vi "GetLoopParameters.vi"(8 "error in (no error)":errorcluster) -> (0 "error out":errorcluster, 3 "This VI":refnum<vi>)   [LabVIEW 2018]
uses:
  <vilib>/Utility/error.llb/DialogType.ctl
  <vilib>/Analysis/1siggen.llb/Ramp Pattern by Samples.vi
  Initialize References/Sequence Globals.vi
  Test Parameter Globals_1.0.0.vi
  <vilib>/Utility/file.llb/Write Delimited Spreadsheet (DBL).vi
  <vilib>/Utility/file.llb/Read Delimited Spreadsheet (string).vi
  <vilib>/Analysis/1siggen.llb/Ramp Pattern by Delta.vi
  Initialize References/Station References Global.vi
  Automated Tests/Tetra WAM/Tetra_Globals.vi
  <vilib>/Utility/file.llb/Write Delimited Spreadsheet (string).vi
  Test Result File Name Global.vi
  <vilib>/Analysis/NI_AALBase.lvlib
panel:
  out "VI Name":string
  out "test_param_path":path
  in  "STOP TEST":bool
  out "#of Iterations(str)":string
  out "Caption.Text":string
  out "Slide":dbl(slide) max=1608.0 step=1.0 scale=0.0..24.0
  out "# of iterations":i32=3
  out "count":dbl
  out "x-y 13":dbl
  out "x-y 12":dbl
  out "x-y 11":dbl
  out "x-y 10":dbl
  out "x-y 9":dbl
  out "x-y 8":dbl
  out "x-y 7":dbl
  out "x-y 6":dbl
  out "x-y 5":dbl
  out "x-y 4":dbl
  out "x-y 3":dbl
  out "x-y 2":dbl
  out "x-y":dbl
  out "Close vi":string="C:\\IdtATE\\Charactorization Tests\\F1200\\SParameter\\F1200_SP_Payload_10.0.0.0.vi"
  out "Test Parameters File":string caption="Test File:"
  out "F-format string":string
  out "Global SN":string="0"
  out "SN":string="15"
  in  "Use auto generated Directory/File Name (T)":bool=TRUE
  out "Test Results File Name":path=path "C:/IdtATE/Results/F1200-ZD_SP_CHAR/F1200-ZD_SP_CHAR_SN_0_131622.csv"
  out "Test Name":string="F1200-ZD_SP_CHAR"
  out "index of element":i32=2
  out "subarray":string[](array[string])=["", "", "TEST NAME", "SN", "", "KEY", "1", "1", "", "KEY", "1", "1", "1", "1", "1", "", "KEY", "3", "3", "-2", "-1", "-1", "-1", "-1", "-1", "", "KEY", "1", "1", "1", "1", "1", "1", "1", "1", "1", "1", "1", "1", "1", "1", "1", "1", "1", "1", "1", "1", "1", "1", "1", "1", "1", "1", "1", "1", "1", "1", "1", "1", "1", "1", "1", "1", "1", "1", "1", "1", "1", "1", "", ""]
  out "Payload vi":string="C:\\IdtATE\\Charactorization Tests\\F1200\\SParameter\\F1200_SP_Payload_10.0.0.0.vi"
  out "Setup vi":string="C:\\IdtATE\\Charactorization Tests\\F1200\\SParameter\\F1200_SP_Setup_10.0.0.0.vi"
  out "Computer Name":string="corpmxl0251xct"
  out "Outputs":string[](array[string])=["GAIN_CODE(8b Word)", "ICC(A)", "S11_30(mag)", "S11_30(ang)", "S21_30(mag)", "S21_30(ang)", "S12_30(mag)", "S12_30(ang)", "S22_30(mag)", "S22_30(ang)", "S11_50(mag)", "S11_50(ang)", "S21_50(mag)", "S21_50(ang)", "S12_50(mag)", "S12_50(ang)", "S22_50(mag)", "S22_50(ang)", "S11_80(mag)", "S11_80(ang)", "S21_80(mag)", "S21_80(ang)", "S12_80(mag)", "S12_80(ang)", "S22_80(mag)", "S22_80(ang)", "S11_100(mag)", "S11_100(ang)", "S21_100(mag)", "S21_100(ang)", "S12_100(mag)", "S12_100(ang)", "S22_100(mag)", "S22_100(ang)", "S11_120(mag)", "S11_120(ang)", "S21_120(mag)", "S21_120(ang)", "S12_120(mag)", "S12_120(ang)", "S22_120(mag)", "S22_120(ang)"]
  out "Output Keys":i32[](array[numeric])=[1, 1, 1, 1, 1, 1, 1, 1, 1, 1, 1, 1, 1, 1, 1, 1, 1, 1, 1, 1, 1, 1, 1, 1, 1, 1, 1, 1, 1, 1, 1, 1, 1, 1, 1, 1, 1, 1, 1, 1, 1, 1]
  out "Last Output Index":i32=68
  out "Loop Info":string[](array[string])=["LIST TEMP:19:-46:79", "LIST VCC:4.75:5:5.25", "RANGE GAIN[-1.25:22]0.25", "846"]
  out "!st Output Index":i32=27
  out "Loop Names":string[](array[string])=["TEMP", "VCC", "GAIN"]
  out "Loop Keys":i32[](array[numeric])=[3, 3, -2, -1, -1, -1, -1, -1]
  out "Const Names":string[](array[string])=["VNA_RECALL (reg)", "CAL_STD (text)", "CAL_FILE (path)", "SOAK_TIME (sec)", "LPT1 Base Address (reg)"]
  out "Const Values":string[](array[string])=["1", "thru", "", "300", "1110"]
  out "Const Keys":i32[](array[numeric])=[1, 1, 1, 1, 1]
  out "Vi Keys":i32[](array[numeric])=[1, 1]
  out "Vi List":string[](array[string])=["C:\\IdtATE\\Charactorization Tests\\F1200\\SParameter\\F1200_SP_Setup_10.0.0.0.vi", "C:\\IdtATE\\Charactorization Tests\\F1200\\SParameter\\F1200_SP_Payload_10.0.0.0.vi"]
  out "# of Const":i32=5
  out "Last Vi Sequence Index":i32=7
  out "1st Vi Sequence Index":i32=6
  out "Loop Values":string[][](array[string])=[["19", "-46", "79", "", "", "", "", "", "", "", "", "", "", "", "", "", "", "", "", "", "", "", "", "", "", "", "", "", "", "", "", "", "", "", "", "", "", "", "", "", "", "", "", "", "", "", "", "", "", "", "", "", "", "", "", "", "", "", "", "", "", "", "", "", "", "", "", "", "", "", "", "", "", "", "", "", "", "", "", "", "", "", "", "", "", "", "", "", "", "", "", "", "", ""], ["4.75", "5", "5.25", "", "", "", "", "", "", "", "", "", "", "", "", "", "", "", "", "", "", "", "", "", "", "", "", "", "", "", "", "", "", "", "", "", "", "", "", "", "", "", "", "", "", "", "", "", "", "", "", "", "", "", "", "", "", "", "", "", "", "", "", "", "", "", "", "", "", "", "", "", "", "", "", "", "", "", "", "", "", "", "", "", "", "", "", "", "", "", "", "", "", ""], ["-1.250000", "-1.000000", "-0.750000", "-0.500000", "-0.250000", "0.000000", "0.250000", "0.500000", "0.750000", "1.000000", "1.250000", "1.500000", "1.750000", "2.000000", "2.250000", "2.500000", "2.750000", "3.000000", "3.250000", "3.500000", "3.750000", "4.000000", "4.250000", "4.500000", "4.750000", "5.000000", "5.250000", "5.500000", "5.750000", "6.000000", "6.250000", "6.500000", "6.750000", "7.000000", "7.250000", "7.500000", "7.750000", "8.000000", "8.250000", "8.500000", "8.750000", "9.000000", "9.250000", "9.500000", "9.750000", "10.000000", "10.250000", "10.500000", "10.750000", "11.000000", "11.250000", "11.500000", "11.750000", "12.000000", "12.250000", "12.500000", "12.750000", "13.000000", "13.250000", "13.500000", "13.750000", "14.000000", "14.250000", "14.500000", "14.750000", "15.000000", "15.250000", "15.500000", "15.750000", "16.000000", "16.250000", "16.500000", "16.750000", "17.000000", "17.250000", "17.500000", "17.750000", "18.000000", "18.250000", "18.500000", "18.750000", "19.000000", "19.250000", "19.500000", "19.750000", "20.000000", "20.250000", "20.500000", "20.750000", "21.000000", "21.250000", "21.500000", "21.750000", "22.000000"]]
  out "Last Const Index":i32=14
  out "1st Loop  Index":i32=17
  out "1st  Const Index":i32=10
types:
  T1 = typedef "DialogType.ctl" = u16
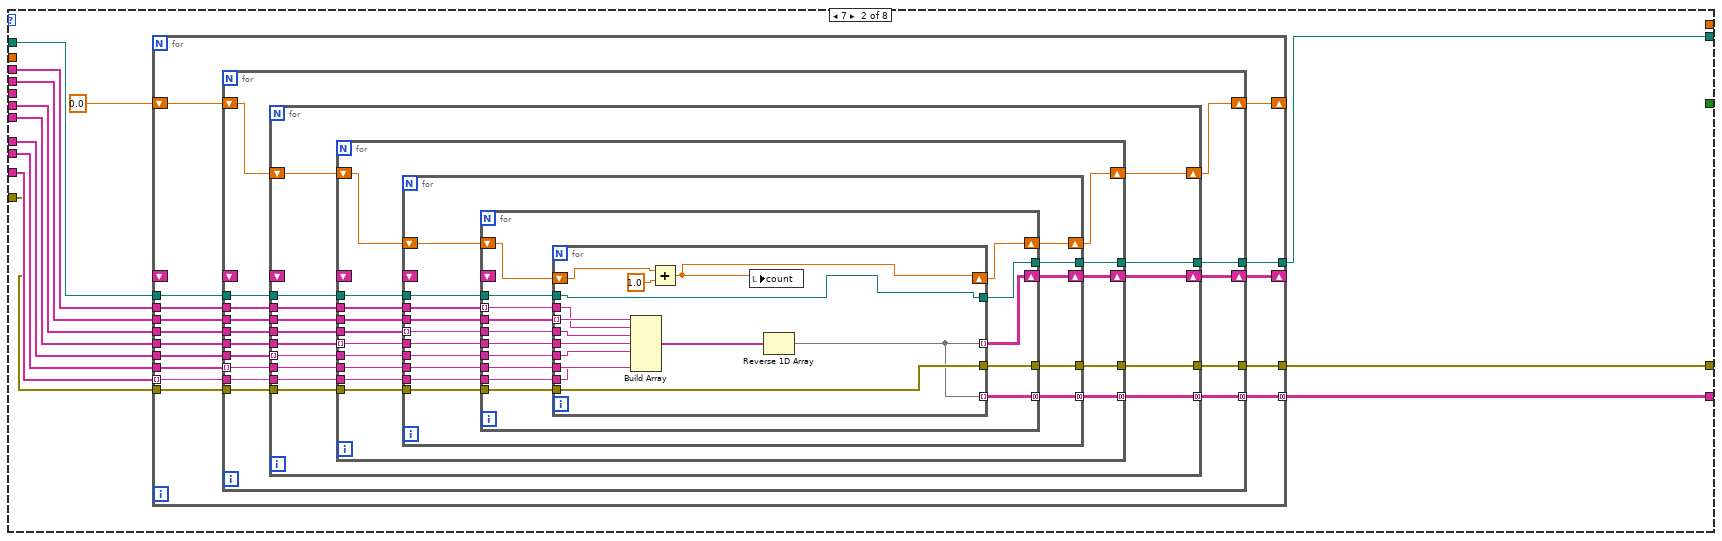
[diagram p3: hidden frame]
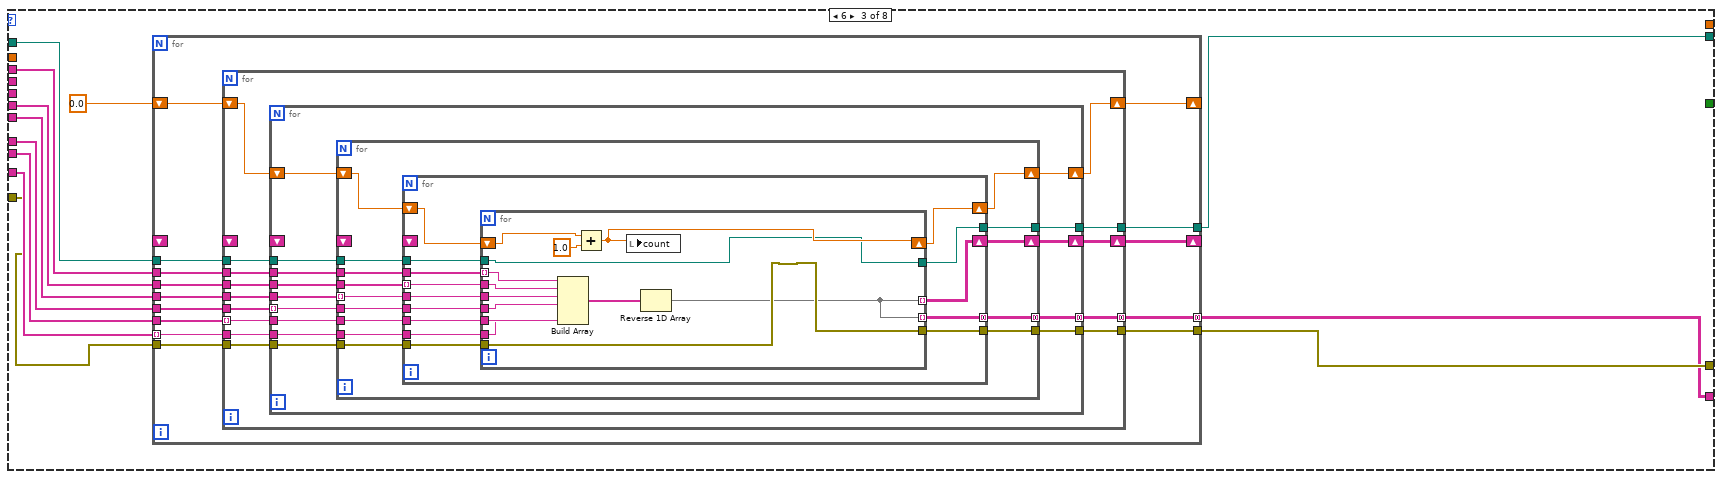
[diagram p4: hidden frame]
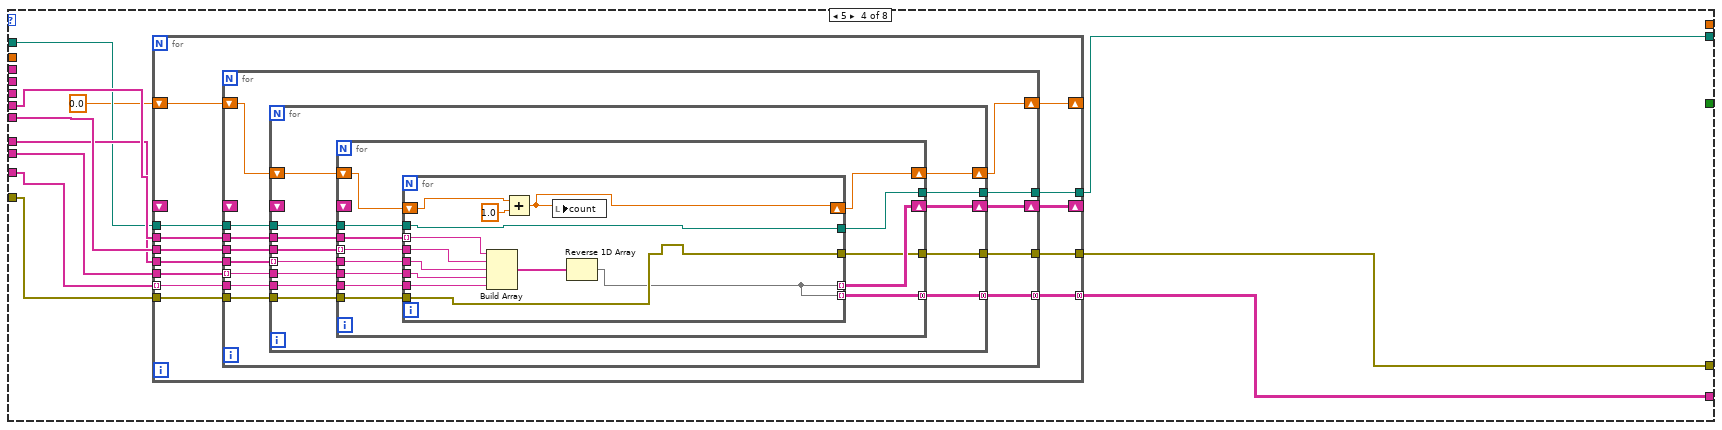
[diagram p5: hidden frame]
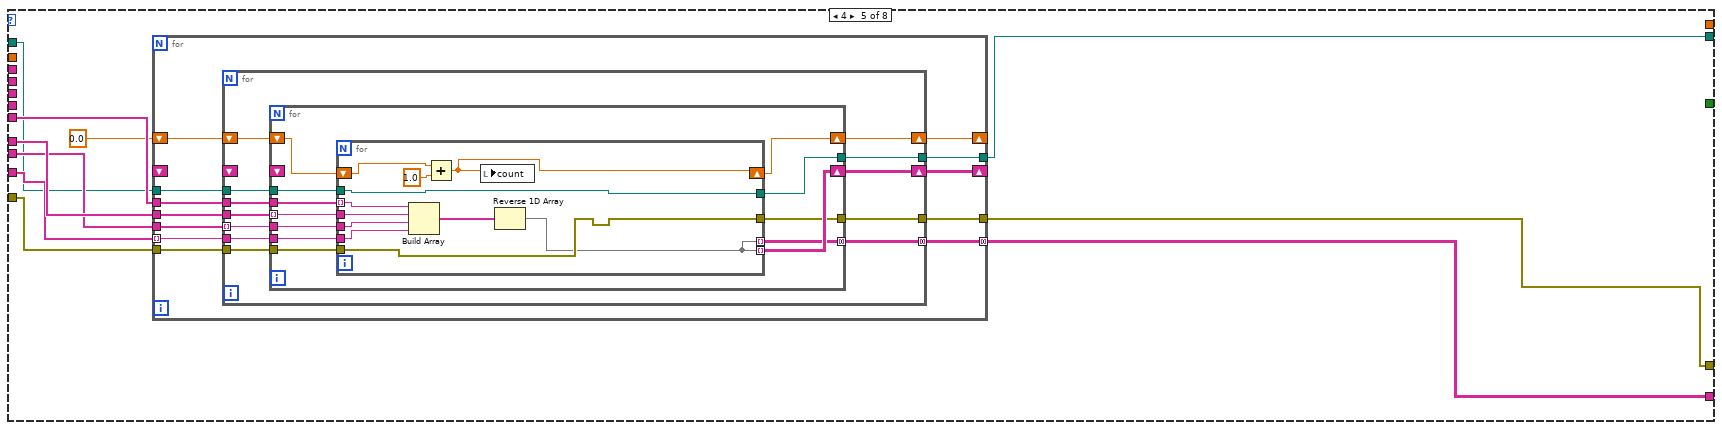
[diagram p6: hidden frame]
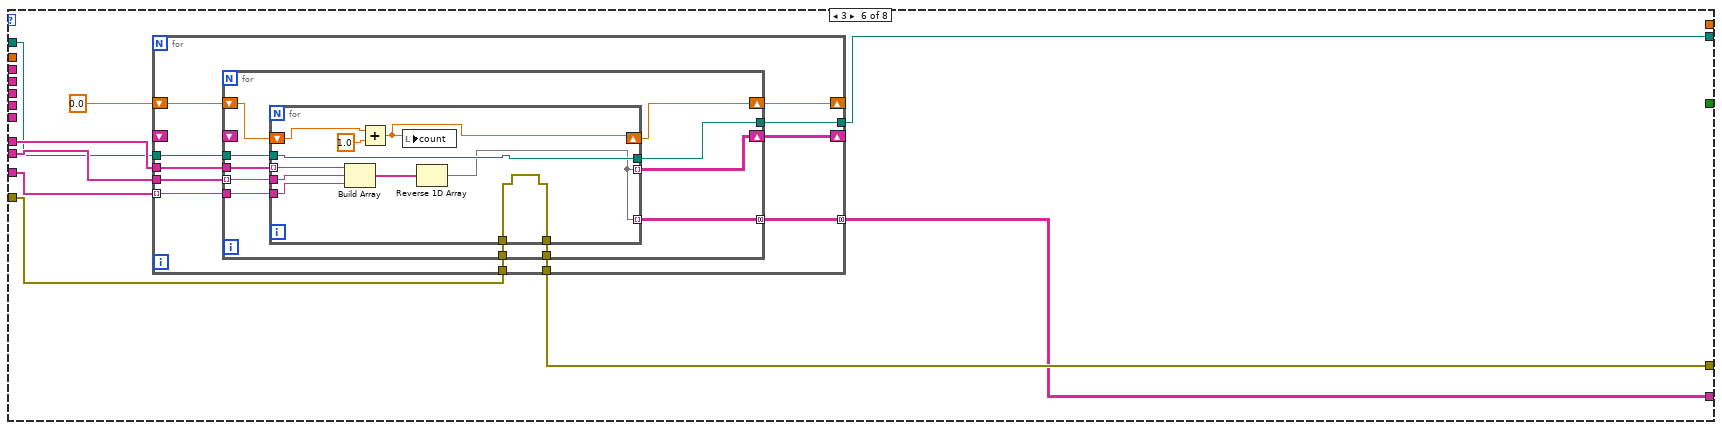
[diagram p7: hidden frame]
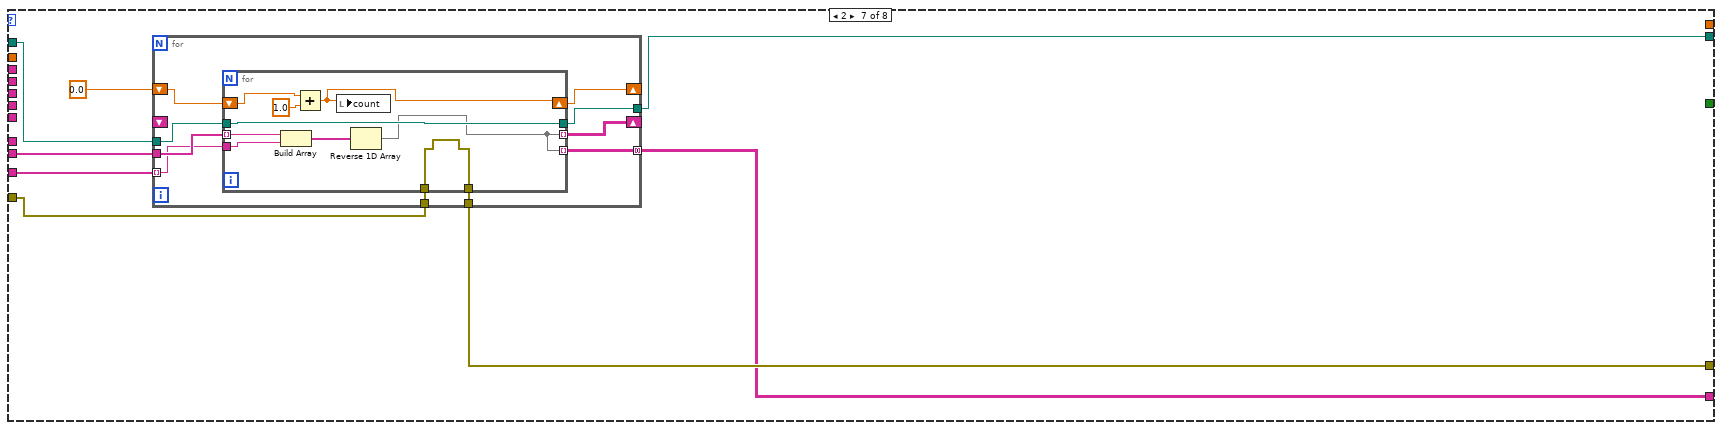
[diagram p8: hidden frame]
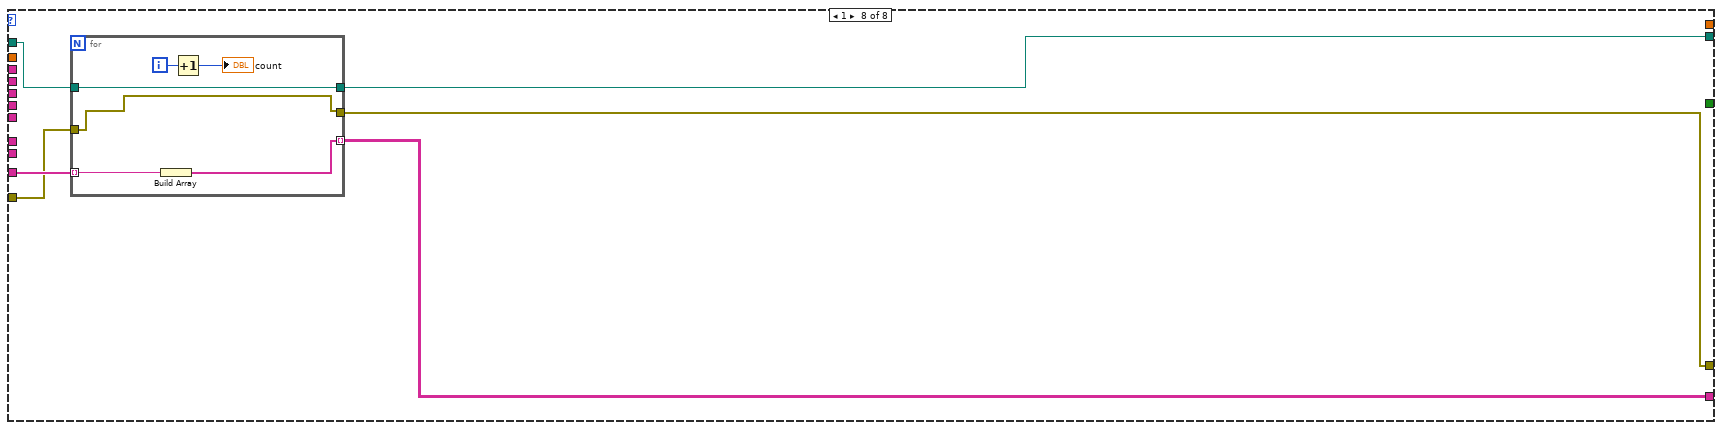
[diagram p9: hidden frame]
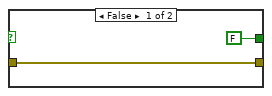
[diagram p13: hidden frame]
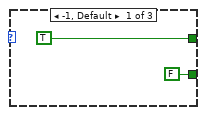
[diagram p16: hidden frame]
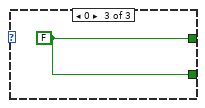
[diagram p17: hidden frame]
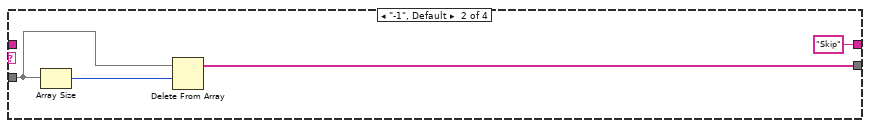
[diagram p18: hidden frame]
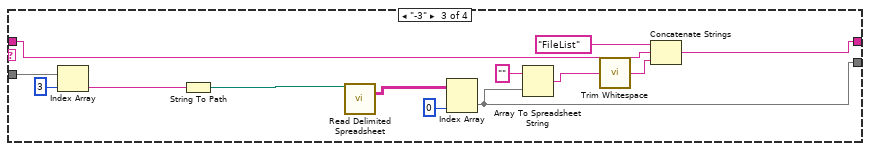
[diagram p19: hidden frame]
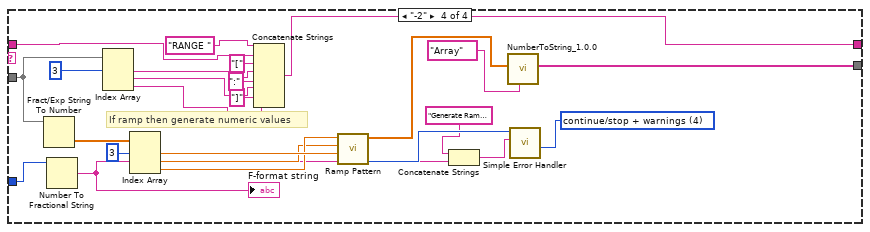
[diagram p20: hidden frame]
diagram:
  n1 = call <vilib>:"High Resolution Relative Seconds.vi"() -> ("relative seconds"=w35:dbl)
  n2 = flat-sequence {
    tunnel: [w86] -> w36
    tunnel: w35 -> [w85]
    tunnel: [w78] -> w19
    tunnel: [w97] -> w61
    tunnel: w36 -> [w117]
    tunnel: [w116] -> w34
    tunnel: w19 -> [w114]
    tunnel: [w108] -> w18
    tunnel: [w141] -> w72
    tunnel: [w139] -> w62
    tunnel: w61 -> [w139]
    tunnel: w34 -> [w137]
    tunnel: [w136] -> w33
    tunnel: w18 -> [w134]
    tunnel: [w131] -> w17
    tunnel: [w155] -> w60
    tunnel: w72 -> [w155]
    tunnel: w62 -> [_]
    tunnel: w33 -> [w149]
    tunnel: [w148] -> w32
    tunnel: w17 -> [w145]
    tunnel: [w144] -> w16
    tunnel: [w231] -> w66
    tunnel: w60 -> [w231]
    tunnel: w32 -> [w222]
    tunnel: [w221] -> w31
    tunnel: w16 -> [w219]
    tunnel: [w219] -> w10
    tunnel: w66 -> [w288]
    tunnel: [w288] -> w70
    tunnel: w31 -> [w276]
    tunnel: [w275] -> w30
    tunnel: [w273] -> w11
    tunnel: w10 -> [w273]
    tunnel: w70 -> [w325]
    tunnel: [w325] -> w71
    tunnel: w30 -> [w321]
    tunnel: [w320] -> w29
    tunnel: [w318] -> w12
    tunnel: w11 -> [w318]
    tunnel: [w358] -> w73
    tunnel: w71 -> [w351]
    tunnel: [w350] -> w69
    tunnel: [w349] -> w68
    tunnel: w29 -> [w348]
    tunnel: [w347] -> w28
    tunnel: [w345] -> w13
    tunnel: w12 -> [w345]
    tunnel: w68 -> [w379]
    tunnel: w69 -> [w380]
    tunnel: w73 -> [w382]
    tunnel: [w377] -> w59
    tunnel: [w382] -> w58
    tunnel: [w381] -> w57
    tunnel: [w377] -> w56
    tunnel: w28 -> [w376]
    tunnel: [w375] -> w27
    tunnel: [w373] -> w14
    tunnel: w13 -> [w373]
    tunnel: w59 -> [w463]
    tunnel: w58 -> [w462]
    tunnel: w57 -> [w461]
    tunnel: w56 -> [w459]
    tunnel: [w463] -> w46
    tunnel: [w462] -> w44
    tunnel: [w461] -> w42
    tunnel: w27 -> [w456]
    tunnel: [w455] -> w26
    tunnel: [w452] -> w15
    tunnel: w14 -> [w452]
    tunnel: w46 -> [w491]
    tunnel: [w491] -> w45
    tunnel: w44 -> [w490]
    tunnel: [w490] -> w43
    tunnel: w42 -> [w489]
    tunnel: [w489] -> w41
    tunnel: w26 -> [w476]
    tunnel: [w475] -> w25
    tunnel: w15 -> [w471]
    tunnel: [w470] -> w9
    tunnel: [w535] -> w65
    tunnel: [w536] -> w67
    tunnel: [w534] -> _
    tunnel: w45 -> [w534]
    tunnel: w43 -> [w536]
    tunnel: w41 -> [w535]
    tunnel: [w533] -> w54
    tunnel: [w532] -> w53
    tunnel: [w531] -> w52
    tunnel: [w530] -> w51
    tunnel: [w529] -> w50
    tunnel: [w528] -> w49
    tunnel: [w527] -> w48
    tunnel: [w526] -> w47
    tunnel: [w521] -> w55
    tunnel: w25 -> [w525]
    tunnel: [w524] -> w22
    tunnel: w9 -> [w519]
    tunnel: [w518] -> w8
    tunnel: [w517] -> w1
    frame #0 {
      n3 = global read "Sequence Globals.vi" "Stop Testing"() -> (w77:bool)
      n4 = control-ref of="Slide"() -> (w81:refnum<vi>)
      n5 = case shown="True" w77 {
        selector: w77 -> [_ w88]
        tunnel: "error in (no error)" -> [w87 w90]
        tunnel: [w87 w89] -> w75
        frame False {
        }
        frame True {
          n6 = global write "Sequence Globals.vi" "Stop Testing"(w88) -> ()
          n7 = flat-sequence {
            tunnel: w88 -> [w94]
            tunnel: [w94] -> w91
            tunnel: w90 -> [w93]
            tunnel: [w92] -> w89
            tunnel: w91 -> [w96]
            frame #0 {
              n8 = control-ref of="This VI"() -> (w95:refnum<vi>)
              n9 = invoke class="VI" method="FP.Close"(reference=w95, error in=w93) -> (error out=w92:errorcluster)  [unwired: 1 in, 2 out]
            }
            frame #1 {
              n10 = Stop(stop? (T)=w96) -> ()
            }
          }
        }
      }
      n11 = property on="Property Node" class="Slide (strict)"(reference=w81, "Caption.Text"="") -> ()  [unwired: 1 in, 2 out]
      n12 = call <vilib>:"High Resolution Relative Seconds.vi"() -> ("relative seconds"=w86:dbl)
      n13 = control-ref of="This VI"() -> (→"This VI":refnum<vi>)
      n14 = local write "STOP TEST"(FALSE ("STOP TEST")) -> ()
      n15 = Subtract(x=w86, y=w85) -> (x-y=→"x-y":dbl)
      n16 = call "Get_computername.vi"("error in (no error)"=w75) -> ("error out"=w78:errorcluster, "Computer Name"=w83:string)  [unwired: 9 in]
      "Computer Name" <- w83
      n17 = global write "Test Parameter Globals_1.0.0.vi" "Computer Name"(w83) -> ()
      "Slide" <- 0.0 ("Slide")
    }
    frame #1 {
      (unwired) path "C:/RageATE/Infrastructure/Test Parameters.tmp" ("file path (dialog if empty)")
      w99 = path "Infrastructure/Test Parameters.tmp" ("file path (dialog if empty)")
      # "Create temp parameter filename"
      n18 = global read "Sequence Globals.vi" "AppSupportPath"() -> (w110:path)
      n19 = global read "Sequence Globals.vi" "IsRuntime?"() -> (w113:bool)
      n20 = Strip Path(path=w99) -> (name=w112:string)  [unwired: 1 out]
      n21 = call <vilib>:"High Resolution Relative Seconds.vi"() -> ("relative seconds"=w116:dbl)
      n22 = global read "Sequence Globals.vi" "DevSupportPath"() -> (w101:path)
      n23 = Build Path(base path=w110, name or relative path=w112) -> (appended path=w111:path)
      n24 = Subtract(x=w116, y=w117) -> (x-y=→"x-y 2":dbl)
      n25 = property class="VI"() -> ("Name"=w104:string)  [unwired: 2 in, 2 out]
      "VI Name" <- w104
      n26 = Strip Path(path=w101) -> (stripped path=w100:path)  [unwired: 1 out]
      n27 = Build Path(base path=w100, name or relative path=w99) -> (appended path=w98:path)
      n28 = Select(t=w111, s=w113, f=w98) -> (s? t:f=w109:path)
      n29 = call-poly <vilib>:"Write Delimited Spreadsheet.vi"("file path (dialog if empty)"=w109, "append to file? (new file:F)"=FALSE, "error in (no error)"=w114, "delimiter (\\t)"="," ("delimiter (\\t)")) -> ("new file path (Not A Path if cancelled)"=w97:path, "error out"=w108:errorcluster)  [unwired: 10 in]
      "test_param_path" <- w97
      n30 = Path To String(path=w97) -> (string=w105:string)
      n31 = Format Into String(format string="%s in VI %s Cant be located", initial string="The File:  ", w105, w104) -> (resulting string=w103:string)  [unwired: 1 in, 1 out]
      n32 = call <vilib>:"Check if File or Folder Exists.vi"("error in (no error)"=w108, "path"=w97) -> ("file or folder exists?"=w102:bool)  [unwired: 7 in, 2 out]
      n33 = case shown="False" w102 {
        tunnel: w103 -> [w120 _]
        frame False {
          n34 = call "Display Message to User2"("Message"=w120) -> ()  [unwired: 9 in, 2 out]
        }
        frame True {
        }
      }
    }
    frame #2 {
      # "Get the test parameter file"
      n35 = global read "Test Parameter Globals_1.0.0.vi" "Test Parameters File"() -> (w123:path)
      n36 = Path To String(path=w123) -> (string=w125:string)
      n37 = property class="VI"() -> ("Name"=w126:string)  [unwired: 2 in, 2 out]
      n38 = call <vilib>:"Check if File or Folder Exists.vi"("path"=w123) -> ("file or folder exists?"=w127:bool)  [unwired: 8 in, 2 out]
      n39 = control-ref of="Test Parameters File"() -> (w133:refnum<vi>)
      n40 = Format Into String(format string="%s in VI %s Cant be located", initial string="The File:  ", w125, w126) -> (resulting string=w121:string)  [unwired: 1 in, 1 out]
      n41 = case shown="False" w127 {
        tunnel: w121 -> [w143 _]
        frame False {
          n42 = call "Display Message to User3"("Message"=w143) -> ()  [unwired: 9 in, 2 out]
        }
        frame True {
        }
      }
      n43 = call <vilib>:"High Resolution Relative Seconds.vi"() -> ("relative seconds"=w136:dbl)
      n44 = Path To String(path=w123) -> (string=w128:string)
      "Test Parameters File" <- w128
      n45 = Concatenate Strings("Test File: " ("string"), w128) -> (w129:string)
      n46 = Subtract(x=w136, y=w137) -> (x-y=→"x-y 3":dbl)
      n47 = call-poly <vilib>:"Read Delimited Spreadsheet.vi"("file path (dialog if empty)"=w123, "error in (no error)"=w134, "transpose? (F)"=FALSE ("transpose (no:F)")) -> ("all rows"=w138:string[][], "error out"=w132:errorcluster)  [unwired: 7 in, 4 out]
      n48 = property class="Str"(reference=w133, error in=w132, "Caption.Text"=w129) -> (error out=w131:errorcluster)  [unwired: 1 out]
      n49 = Delete From Array(array=w138, index (col)=0 ("disabled index (col)")) -> (array with subset deleted=w141:string[][])  [unwired: 2 in, 1 out]
    }
    frame #3 {
      w161 = 0 ("disabled index (col)")
      # "Generate Indices with a keyword search"
      n50 = To Upper Case(1:w155) -> (0:w164:string[][])
      n51 = call <vilib>:"High Resolution Relative Seconds.vi"() -> ("relative seconds"=w148:dbl)
      n52 = Subtract(x=w148, y=w149) -> (x-y=→"x-y 4":dbl)
      n53 = To Upper Case(1:"VI Sequence" ("element")) -> (0:w193:string)
      n54 = To Upper Case(1:"End Parameters" ("string")) -> (0:w175:string)
      n55 = To Upper Case(1:"Loop Parameters" ("element")) -> (0:w150:string)
      n56 = To Upper Case(1:"Outputs" ("string")) -> (0:w178:string)
      n57 = To Upper Case(1:"Input Constants" ("element")) -> (0:w191:string)
      n58 = Index Array(array=w155, index (col)=1 ("disabled index (col)")) -> (element=w165:string[])  [unwired: 1 in]
      n59 = Index Array(array=w164, index (col)=w161) -> (element=w146:string[])  [unwired: 1 in]
      "subarray" <- w146
      n60 = To Upper Case(1:w165) -> (0:w194:string[])
      n61 = To Upper Case(1:w165) -> (0:w176:string[])
      n62 = To Upper Case(1:w165) -> (0:w179:string[])
      n63 = To Upper Case(1:w165) -> (0:w166:string[])
      n64 = To Upper Case(1:w165) -> (0:w192:string[])
      n65 = To Upper Case(1:"TEST NAME" ("element")) -> (0:w151:string)
      n66 = To Upper Case(1:"SN" ("element")) -> (0:w157:string)
      n67 = Add(x=w161, y=1) -> (x+y=w154:i32)
      n68 = To Upper Case(1:w146) -> (0:w163:string[])
      n69 = Search 1D Array(1D array=w194, element=w193) -> (index of element=w183:i32)  [unwired: 1 in]
      n70 = Search 1D Array(1D array=w176, element=w175) -> (index of element=w173:i32)  [unwired: 1 in]
      n71 = Search 1D Array(1D array=w179, element=w178) -> (index of element=w170:i32)  [unwired: 1 in]
      n72 = Search 1D Array(1D array=w166, element=w191) -> (index of element=w181:i32)  [unwired: 1 in]
      n73 = Search 1D Array(1D array=w192, element=w150) -> (index of element=w182:i32)  [unwired: 1 in]
      n74 = To Upper Case(1:w146) -> (0:w156:string[])
      n75 = Search 1D Array(1D array=w163, element=w151) -> (index of element=w162:i32)  [unwired: 1 in]
      "index of element" <- w162
      n76 = Search 1D Array(1D array=w156, element=w157) -> (index of element=w153:i32)  [unwired: 1 in]
      n77 = Build Array(w183, w182, w181) -> (w180:i32[])
      n78 = Add(x=1, y=w183) -> (x+y=→"1st Vi Sequence Index":i32)
      n79 = Subtract(x=w173, y=2) -> (x-y=→"Last Output Index":i32)
      n80 = Add(x=w170, y=1) -> (x+y=→"!st Output Index":i32)
      n81 = Subtract(x=w181, y=2 ("x")) -> (x-y=→"Last Vi Sequence Index":i32)
      n82 = Add(x=w181, y=1) -> (x+y=w197:i32)
      "1st  Const Index" <- w197
      n83 = Add(x=0, y=w182) -> (x+y=w202:i32)
      n84 = for {
        tunnel: w180 -> [w212] mode=indexing
        tunnel: w145 -> [w208]
        tunnel: [w207] -> w144
        # "Check for Spreadsheet Errors"
        n85 = Equal?(x=w212, y=-1) -> (x = y?=w210:bool)
        n86 = case shown="True" w210 {
          tunnel: [FALSE ("OK") w217] -> w209
          tunnel: w208 -> [w213 w216]
          tunnel: [w213 w215] -> w207
          frame False {
          }
          frame True {
            n87 = call "Display Message to User"("error in (no error)"=w216) -> ("error out"=w215:errorcluster, "OK"=w217:bool)  [unwired: 9 in]
          }
        }
        n88 = Stop(stop? (T)=w209) -> ()
      }
      n89 = Subtract(x=w202, y=2) -> (x-y=w185:i32)
      "Last Const Index" <- w185
      n90 = Add(x=1, y=w202) -> (x+y=→"1st Loop  Index":i32)
      n91 = Subtract(x=w185, y=w197) -> (x-y=w199:i32)
      n92 = Index Array(array=w155, index (row)=w162, index (col)=w154) -> (element=w159:string)
      "Test Name" <- w159
      n93 = Index Array(array=w155, index (row)=w153, index (col)=w154) -> (element=→"SN":string)
      n94 = Add(x=w199, y=1) -> (x+y=→"# of Const":i32)
      n95 = global write "Test Parameter Globals_1.0.0.vi" "Test Name"(w159) -> ()
    }
    frame #4 {
      n96 = local read "Last Output Index"() -> (w226:i32)
      n97 = local read "!st Output Index"() -> (w227:i32)
      n98 = call <vilib>:"High Resolution Relative Seconds.vi"() -> ("relative seconds"=w221:dbl)
      n99 = Subtract(x=w221, y=w222) -> (x-y=→"x-y 5":dbl)
      n100 = Subtract(x=w226, y=w227) -> (x-y=w230:i32)
      n101 = Add(x=w230, y=1) -> (x+y=w228:i32)
      n102 = call-poly <vilib>:"Ramp Pattern.vi"("start"=w227, "end"=w226, "samples"=w228) -> ("Ramp Pattern"=w232:dbl[])  [unwired: 7 in, 1 out]
      n103 = for {
        tunnel: w231 -> [w249]
        tunnel: w232 -> [w242] mode=indexing
        tunnel: [w248] -> w225 mode=indexing
        tunnel: [w243] -> w218 mode=indexing
        tunnel: [w240] -> w224 mode=indexing
        n104 = Index Array(array=w249, index (row) #1=w242, index (col) #1=0 ("disabled index (col)"), index (row) #2=w242, index (col) #2=1 ("disabled index (col)"), index (row) #3=w242, index (col) #3=2 ("disabled index (col)")) -> (element #1=w245:string, element #2=w248:string, element #3=w240:string)
        n105 = Fract/Exp String To Number(string=w245, default (0 dbl)=0 ("default (0 DBL)")) -> (number=w243:i32)  [unwired: 2 in, 1 out]
      }
      "Output Keys" <- w218
      n106 = for {
        tunnel: w225 -> [w239] mode=indexing
        tunnel: w224 -> [w237] mode=indexing
        tunnel: [w235] -> w223 mode=indexing if=w233
        tunnel: w218 -> [w234] mode=indexing
        n107 = Concatenate Strings(w239, "(" ("string"), w237, ")" ("string")) -> (w235:string)
        n108 = Not Equal To 0?(x=w234) -> (x != 0?=w233:bool)
      }
      "Outputs" <- w223
    }
    frame #5 {
      # "Vi Keys\n0 = Dont run\n1= Run /FP open\n-1= Run /FP closed"
      n109 = local read "Last Vi Sequence Index"() -> (w292:i32)
      n110 = local read "1st Vi Sequence Index"() -> (w282:i32)
      n111 = Subtract(x=w292, y=w282) -> (x-y=w291:i32)
      n112 = call <vilib>:"High Resolution Relative Seconds.vi"() -> ("relative seconds"=w275:dbl)
      n113 = Add(x=w291, y=1) -> (x+y=w290:i32)
      n114 = Subtract(x=w275, y=w276) -> (x-y=→"x-y 6":dbl)
      n115 = call-poly <vilib>:"Ramp Pattern.vi"("start"=w282, "end"=w292, "samples"=w290) -> ("Ramp Pattern"=w287:dbl[])  [unwired: 7 in, 1 out]
      n116 = for {
        tunnel: w288 -> [w317]
        tunnel: w287 -> [w315] mode=indexing
        tunnel: [w316] -> w286 mode=indexing
        tunnel: [w310] -> w284 mode=indexing
        n117 = Index Array(array=w317, index (row) #1=w315, index (col) #1=0 ("disabled index (col)"), index (row) #2=w315, index (col) #2=2 ("disabled index (col)")) -> (element #1=w312:string, element #2=w316:string)
        n118 = Fract/Exp String To Number(string=w312, default (0 dbl)=0 ("default (0 DBL)")) -> (number=w310:i32)  [unwired: 2 in, 1 out]
      }
      "Vi List" <- w286
      "Vi Keys" <- w284
      n119 = global read "Sequence Globals.vi" "AppSupportPath"() -> (w261:path)
      n120 = global read "Sequence Globals.vi" "IsRuntime?"() -> (w259:bool)
      n121 = for {
        tunnel: w284 -> [w304] mode=indexing
        tunnel: [w303] -> w283 mode=indexing
        tunnel: [w302] -> w277 mode=indexing
        n122 = case shown="1" w304 {
          tunnel: [TRUE TRUE w309] -> w303
          tunnel: [FALSE TRUE w309] -> w302
          frame -1, Default {
          }
          frame 1 {
          }
          frame 0 {
            w309 = FALSE
          }
        }
      }
      n123 = Index Array(array=w286) -> (element #1=w285:string, element #2=w266:string, element #3=w281:string)  [unwired: 3 in]
      n124 = String To Path(string=w285) -> (path=w270:path)
      n125 = String To Path(string=w266) -> (path=w264:path)
      n126 = String To Path(string=w281) -> (path=w260:path)
      n127 = global write "Test Parameter Globals_1.0.0.vi" "Payload Path"(w264) -> ()
      n128 = global write "Test Parameter Globals_1.0.0.vi" "Close vi"(w260) -> ()
      n129 = global write "Test Parameter Globals_1.0.0.vi" "Setup Path"(w270) -> ()
      n130 = Strip Path(path=w260) -> (name=w262:string)  [unwired: 1 out]
      n131 = Strip Path(path=w270) -> (name=w271:string)  [unwired: 1 out]
      n132 = Build Path(base path=w261, name or relative path=w262) -> (appended path=w263:path)
      n133 = Strip Path(path=w264) -> (name=w268:string)  [unwired: 1 out]
      n134 = Build Path(base path=w261, name or relative path=w271) -> (appended path=w272:path)
      n135 = Build Path(base path=w261, name or relative path=w268) -> (appended path=w267:path)
      n136 = Select(t=w263, s=w259, f=w260) -> (s? t:f=w255:path)
      n137 = Index Array(array=w283) -> (element #1=w254:bool, element #2=w253:bool, element #3=w252:bool)  [unwired: 3 in]
      n138 = Path To String(path=w255) -> (string=→"Close vi":string)
      n139 = Index Array(array=w277) -> (element #1=w280:bool, element #2=w279:bool, element #3=w278:bool)  [unwired: 3 in]
      n140 = Select(t=w272, s=w259, f=w270) -> (s? t:f=w257:path)
      n141 = Select(t=w267, s=w259, f=w264) -> (s? t:f=w256:path)
      n142 = Path To String(path=w256) -> (string=→"Payload vi":string)
      n143 = Path To String(path=w257) -> (string=→"Setup vi":string)
      n144 = global write "Test Parameter Globals_1.0.0.vi" "Close vi"(w255) -> ()
      n145 = global write "Test Parameter Globals_1.0.0.vi" "Show Setup FP"(w280) -> ()
      n146 = global write "Test Parameter Globals_1.0.0.vi" "Show Payload FP"(w279) -> ()
      n147 = global write "Test Parameter Globals_1.0.0.vi" "Run Setup vi"(w254) -> ()
      n148 = global write "Test Parameter Globals_1.0.0.vi" "Run Payload vi"(w253) -> ()
      n149 = global write "Test Parameter Globals_1.0.0.vi" "Show Close FP"(w278) -> ()
      n150 = global write "Test Parameter Globals_1.0.0.vi" "Payload Path"(w256) -> ()
      n151 = global write "Test Parameter Globals_1.0.0.vi" "Run Close vi"(w252) -> ()
      n152 = global write "Test Parameter Globals_1.0.0.vi" "Setup Path"(w257) -> ()
      n153 = Build Array(w254, w253, w252) -> (w251:bool[])
      n154 = Build Array(w257, w256, w255) -> (w250:path[])
      n155 = for {
        tunnel: w251 -> [w297] mode=indexing
        tunnel: w250 -> [w294] mode=indexing
        n156 = local read "VI Name"() -> (w295:string)
        n157 = Format Into String(format string="The File < %s > cant be found\nVI : %s", w294, w295) -> (resulting string=w293:string)  [unwired: 2 in, 1 out]
        n158 = case shown="True" w297 {
          tunnel: w294 -> [_ w300]
          tunnel: w293 -> [_ w299]
          frame False {
          }
          frame True {
            n159 = call <vilib>:"Check if File or Folder Exists.vi"("path"=w300) -> ("file or folder exists?"=w298:bool)  [unwired: 8 in, 2 out]
            n160 = case shown="False" w298 {
              tunnel: w299 -> [w301 _]
              frame False {
                n161 = call "Display Message to User4"("Message"=w301) -> ()  [unwired: 9 in, 2 out]
              }
              frame True {
              }
            }
          }
        }
      }
    }
    frame #6 {
      # "Get the Input Constants"
      n162 = local read "Last Const Index"() -> (w327:i32)
      n163 = local read "1st  Const Index"() -> (w326:i32)
      n164 = local read "# of Const"() -> (w328:i32)
      n165 = call <vilib>:"High Resolution Relative Seconds.vi"() -> ("relative seconds"=w320:dbl)
      n166 = Subtract(x=w320, y=w321) -> (x-y=→"x-y 7":dbl)
      n167 = call-poly <vilib>:"Ramp Pattern.vi"("start"=w326, "end"=w327, "samples"=w328) -> ("Ramp Pattern"=w329:dbl[])  [unwired: 7 in, 1 out]
      n168 = for {
        tunnel: w325 -> [w344]
        tunnel: w329 -> [w337] mode=indexing
        tunnel: [w341] -> w324 mode=indexing
        tunnel: [w335] -> w323 mode=indexing
        tunnel: [w330] -> w322 mode=indexing
        n169 = Index Array(array=w344, index (row) #1=w337, index (col) #1=0 ("disabled index (col)"), index (row) #2=w337, index (col) #2=1 ("disabled index (col)"), index (row) #3=w337, index (col) #3=2 ("disabled index (col)"), index (row) #4=w337, index (col) #4=3 ("disabled index (col)")) -> (element #1=w340:string, element #2=w334:string, element #3=w332:string, element #4=w335:string)
        n170 = Concatenate Strings(w334, " (" ("string"), w332, ")" ("string")) -> (w330:string)
        n171 = Fract/Exp String To Number(string=w340, default (0 dbl)=0 ("default (0 DBL)")) -> (number=w341:i32)  [unwired: 2 in, 1 out]
      }
      "Const Keys" <- w324
      "Const Values" <- w323
      "Const Names" <- w322
    }
    frame #7 {
      # "Get the 8 Loops"
      # "Adjust the array size by counting -1 keys"
      n172 = local read "1st Loop  Index"() -> (w354:i32)
      n173 = Add(x=7.0 ("end"), y=w354) -> (x+y=w356:dbl)
      n174 = call-poly <vilib>:"Ramp Pattern.vi"("start"=w354, "end"=w356, "samples"=8 ("x")) -> ("Ramp Pattern"=w353:dbl[])  [unwired: 7 in, 1 out]
      n175 = call <vilib>:"High Resolution Relative Seconds.vi"() -> ("relative seconds"=w347:dbl)
      n176 = Subtract(x=w347, y=w348) -> (x-y=→"x-y 8":dbl)
      n177 = for {
        tunnel: w351 -> [w362]
        tunnel: w353 -> [w361] mode=indexing
        tunnel: [w366] -> w352 mode=indexing
        tunnel: [w364] -> w349 mode=indexing
        tunnel: [w360] -> w350 mode=indexing
        n178 = Index Array(array=w362, index (row) #1=w361, index (col) #1=0 ("disabled index (col)"), index (row) #2=w361, index (col) #2=1 ("disabled index (col)"), index (row) #3=w361) -> (element #1=w363:string, element #2=w364:string, element #3=w360:string[])  [unwired: 1 in]
        n179 = Fract/Exp String To Number(string=w363, default (0 dbl)=0 ("default (0 DBL)")) -> (number=w366:i32)  [unwired: 2 in, 1 out]
      }
      "Loop Keys" <- w352
      n180 = for {
        tunnel: [w371] -> w359 mode=indexing
        tunnel: w352 -> [w369] mode=indexing
        n181 = Not Equal?(x=w369, y=-1.0) -> (x != y?=w372:bool)
        n182 = Boolean To (0,1)(Boolean=w372) -> (0, 1=w371:i16)
      }
      n183 = Add Array Elements(numeric array=w359) -> (sum=w358:i16)
    }
    frame #8 {
      n184 = for {
        N: w382 -> [_]
        tunnel: w380 -> [w387] mode=indexing
        tunnel: [w386] -> w377 mode=indexing
        tunnel: w379 -> [w385] mode=indexing
        tunnel: [w385] -> w378 mode=indexing
        tunnel: [w384] -> w381 mode=indexing
        i -> [w383]
        n185 = stacked-sequence {
          tunnel: w387 -> [w394]
          tunnel: [w392] -> w386
          tunnel: w385 -> [w390]
          tunnel: [w389] -> w384
          tunnel: w383 -> [w388]
          frame #0 {
            n186 = Index Array(array=w394, index=0) -> (element=w391:string)
            n187 = case shown="\"1\".." w391 {
              selector: w391 -> [w401 _ _ _]
              tunnel: w394 -> [w402 w413 w426 w446]
              tunnel: [w395 w411 w420 w444] -> w392
              tunnel: [w399 "Skip" w421 w440] -> w389
              tunnel: w390 -> [w398 _ w418 w432]
              tunnel: w388 -> [_ _ _ w430]
              frame "1".. {
                n188 = Fract/Exp String To Number(string=w401) -> (number=w400:dbl)  [unwired: 3 in, 1 out]
                n189 = for {
                  N: w400 -> [_]
                  tunnel: w402 -> [w409]
                  tunnel: [w403] -> w395 mode=indexing
                  tunnel: [w404] -> w397 mode=indexing
                  i -> [w408]
                  n190 = Add(x=3, y=w408) -> (x+y=w406:i32)
                  n191 = Index Array(array=w409, index=w406) -> (element=w403:string)
                  n192 = Concatenate Strings(":" ("string"), w403) -> (w404:string)
                }
                n193 = Concatenate Strings("LIST ", w398, w397) -> (w399:string)
              }
              frame "-1", Default {
                n194 = Array Size(array=w413) -> (size(s)=w412:i32)
                n195 = Delete From Array(array=w413, length=w412) -> (array with subset deleted=w411:string[])  [unwired: 1 in, 1 out]
              }
              frame "-3" {
                n196 = Index Array(array=w426, index=3) -> (element=w424:string)
                n197 = String To Path(string=w424) -> (path=w425:path)
                n198 = call-poly <vilib>:"Read Delimited Spreadsheet.vi"("file path (dialog if empty)"=w425) -> ("all rows"=w414:string[][])  [unwired: 9 in, 5 out]
                n199 = Index Array(array=w414, index (col)=0 ("disabled index (col)")) -> (element=w420:string[])  [unwired: 1 in]
                n200 = Array To Spreadsheet String(array=w420, 3:"" ("format string")) -> (spreadsheet string=w416:string)  [unwired: 1 in]
                n201 = call <vilib>:"Trim Whitespace.vi"("string"=w416) -> ("trimmed string"=w415:string)  [unwired: 1 in]
                n202 = Concatenate Strings("FileList", w418, w415) -> (w421:string)
              }
              frame "-2" {
                w431 = T1 4 items=["no dialog", "OK message", "continue or stop message", "OK message + warnings", "continue/stop + warnings"] ("type of dialog (OK msg:1)")
                # "If ramp then generate numeric values"
                n203 = Fract/Exp String To Number(string=w446) -> (number=w451:dbl[])  [unwired: 3 in, 1 out]
                n204 = Number To Fractional String(number=w430) -> (F-format string=w428:string)  [unwired: 3 in]
                "F-format string" <- w428
                n205 = Index Array(array=w446, index #1=3 ("index")) -> (element #1=w438:string, element #2=w436:string, element #3=w434:string)  [unwired: 2 in]
                n206 = Index Array(array=w451, index #1=3 ("index")) -> (element #1=w450:dbl, element #2=w448:dbl, element #3=w449:dbl)  [unwired: 2 in]
                n207 = Concatenate Strings("RANGE " ("string"), w432, "[" ("string"), w438, ":" ("string"), w436, "]" ("string"), w434) -> (w440:string)
                n208 = call-poly <vilib>:"Ramp Pattern.vi"("start"=w450, "end"=w448, "delta"=w449) -> ("error"=w441:i32, "Ramp Pattern"=w443:dbl[])  [unwired: 6 in, 1 out]
                n209 = Concatenate Strings("Generate Ramp Pattern\nCheck Spreadsheet Ramp values at Index " ("error source (\" \")"), w428) -> (w427:string)
                n210 = call "NumberToString_1.0.0.vi"("Input Select"="Array", "Num (ary)"=w443) -> ("F-format string (ary)"=w444:string[])  [unwired: 8 in, 1 out]
                n211 = call <vilib>:"Simple Error Handler.vi"("error code (no error:0)"=w441, "error source (\" \")"=w427, "type of dialog (OK msg:1)"=w431) -> ()  [unwired: 2 in, 5 out]
              }
            }
          }
        }
      }
      "Loop Values" <- w377
      "Loop Names" <- w378
      n212 = call <vilib>:"High Resolution Relative Seconds.vi"() -> ("relative seconds"=w375:dbl)
      n213 = Subtract(x=w375, y=w376) -> (x-y=→"x-y 9":dbl)
    }
    frame #9 {
      n214 = global write "Test Parameter Globals_1.0.0.vi" "Test Parameters"(w459) -> ()
      n215 = local read "Const Values"() -> (w457:string[])
      n216 = local read "Loop Names"() -> (w453:string[])
      n217 = local read "Outputs"() -> (w460:string[])
      n218 = global write "Test Parameter Globals_1.0.0.vi" "Input Constants Out"(w457) -> ()
      n219 = call <vilib>:"High Resolution Relative Seconds.vi"() -> ("relative seconds"=w455:dbl)
      n220 = global write "Test Parameter Globals_1.0.0.vi" "Loop Names"(w453) -> ()
      n221 = Insert Into Array(array=w453, new element=w460) -> (w458:string[])  [unwired: 1 in]
      n222 = Subtract(x=w455, y=w456) -> (x-y=→"x-y 10":dbl)
      n223 = global write "Test Parameter Globals_1.0.0.vi" "Column Headers Global"(w458) -> ()
    }
    frame #10 {
      n224 = global read "Test Parameter Globals_1.0.0.vi" "User Prompt for SN (T)"() -> (w473:bool)
      n225 = call <vilib>:"High Resolution Relative Seconds.vi"() -> ("relative seconds"=w475:dbl)
      n226 = case shown="False" w473 {
        tunnel: [w492 w493] -> w479
        frame False {
          n227 = local read "SN"() -> (w492:string)
        }
        frame True {
          n228 = global read "Test Parameter Globals_1.0.0.vi" "Global SN"() -> (w493:string)
        }
      }
      "Global SN" <- w479
      n229 = Subtract(x=w475, y=w476) -> (x-y=→"x-y 11":dbl)
      n230 = global read "Test Parameter Globals_1.0.0.vi" "LOT ID"() -> (w465:string)
      n231 = global read "Station References Global.vi" "Test Station Information"() -> (w481:string)
      n232 = global read "Tetra_Globals.vi" "TestBench_ID"() -> (w468:string)
      n233 = global write "Test Parameter Globals_1.0.0.vi" "Global SN"(w479) -> ()
      n234 = local read "Payload vi"() -> (w482:string)
      n235 = local read "Setup vi"() -> (w485:string)
      n236 = Concatenate Strings(w479, "_" ("string"), w465) -> (w467:string)
      n237 = global read "Tetra_Globals.vi" "-ssid"() -> (w464:string)
      n238 = local read "Test Parameters File"() -> (w477:string)
      n239 = local read "Computer Name"() -> (w487:string)
      n240 = local read "Const Names"() -> (w484:string[])
      n241 = local read "Const Values"() -> (w483:string[])
      n242 = local read "Const Keys"() -> (w469:i32[])
      n243 = local read "Test Name"() -> (w486:string)
      n244 = call "GenerateHeaderAndFilename.vi"("Computer"=w487, "Instrument Information"=w481, "Test Name"=w486, "Payload vi Name"=w482, "Ssid"=w464, "Setup vi Name"=w485, "Test Parameter File Name"=w477, "Input Constants Keys"=w469, "SN"=w467, "Input Constants Names"=w484, "BenchId"=w468, "Input Constants Values"=w483) -> ("Header"=w472:string[], "Filename Path"=w480:path)  [unwired: 6 in]
      n245 = case shown="False" "Use auto generated Directory/File Name (T)" {
        tunnel: [w498 w514] -> w478
        tunnel: w480 -> [_ w509]
        tunnel: w472 -> [w497 w508]
        tunnel: w471 -> [w495 w506]
        tunnel: [w494 w505] -> w470
        frame False {
          n246 = Insert Into Array(array=w497, new element="" ("new element/subarray")) -> (w496:string[])  [unwired: 1 in]
          n247 = call-poly <vilib>:"Write Delimited Spreadsheet.vi"("1D data"=w496, "error in (no error)"=w495, "transpose? (no:F)"=TRUE, "delimiter (\\t)"="," ("delimiter (\\t)")) -> ("new file path (Not A Path if cancelled)"=w498:path, "error out"=w494:errorcluster)  [unwired: 10 in]
          n248 = call-poly <vilib>:"Write Delimited Spreadsheet.vi"("file path (dialog if empty)"=w498, "append to file? (new file:F)"=TRUE, "transpose? (no:F)"=TRUE, "delimiter (\\t)"="," ("delimiter (\\t)")) -> ()  [unwired: 10 in, 2 out]
        }
        frame True {
          n249 = Insert Into Array(array=w508, new element="" ("new element/subarray")) -> (w507:string[])  [unwired: 1 in]
          n250 = call-poly <vilib>:"Write Delimited Spreadsheet.vi"("file path (dialog if empty)"=w509, "1D data"=w507, "error in (no error)"=w506, "transpose? (no:F)"=TRUE, "delimiter (\\t)"="," ("delimiter (\\t)")) -> ("new file path (Not A Path if cancelled)"=w514:path, "error out"=w505:errorcluster)  [unwired: 9 in]
          n251 = call-poly <vilib>:"Write Delimited Spreadsheet.vi"("file path (dialog if empty)"=w514, "append to file? (new file:F)"=TRUE, "transpose? (no:F)"=TRUE, "delimiter (\\t)"="," ("delimiter (\\t)")) -> ()  [unwired: 10 in, 2 out]
        }
      }
      "Test Results File Name" <- w478
      n252 = global write "Test Result File Name Global.vi" "Test Results File Name"(w478) -> ()
    }
    frame #11 {
      w522 = "Generating Test Parameters File :"
      n253 = call "CleanUpArray.vi"("Ary In"=w534) -> ("Count"=w521:dbl, "Ary 1"=w526:string[], "Ary 2"=w527:string[], "Ary 3"=w528:string[], "Ary 4"=w529:string[], "Ary 5"=w530:string[], "Ary 6"=w531:string[], "Ary 7"=w532:string[], "Ary 8"=w533:string[])  [unwired: 18 in]
      "# of iterations" <- w521
      n254 = call <vilib>:"High Resolution Relative Seconds.vi"() -> ("relative seconds"=w524:dbl)
      n255 = Subtract(x=w524, y=w525) -> (x-y=→"x-y 12":dbl)
      n256 = global write "Test Parameter Globals_1.0.0.vi" "# of iterations"(w521) -> ()
      n257 = property on="Slide" class="Slide (strict)"(error in=w519, "Scale.Maximum"=w521, "Caption.Text"=w522) -> (error out=w518:errorcluster)  [unwired: 1 in, 1 out]
      n258 = Number To Decimal String(number=w521) -> (decimal integer string=→"#of Iterations(str)":string)  [unwired: 1 in]
      n259 = local read "test_param_path"() -> (w517:path)
      "Caption.Text" <- w522
    }
  }
  n260 = Array Size(array=w65) -> (size(s)=w64:i32)
  n261 = Number To Fractional String(number=w55, precision (6)=i16 0) -> (F-format string=w39:string)  [unwired: 2 in]
  n262 = case shown="8, Default" w67 {
    tunnel: w54 -> [w552 _ _ _ _ _ _ _]
    tunnel: w53 -> [w551 w707 _ _ _ _ _ _]
    tunnel: w52 -> [w550 w706 w823 _ _ _ _ _]
    tunnel: w51 -> [w549 w705 w822 w917 _ _ _ _]
    tunnel: w50 -> [w548 w704 w821 w916 w991 _ _ _]
    tunnel: w49 -> [w547 w703 w820 w915 w990 w1047 _ _]
    tunnel: w48 -> [w546 w702 w819 w914 w989 w1046 w1087 _]
    tunnel: w47 -> [w545 w701 w818 w913 w988 w1045 w1086 w1112]
    tunnel: [w544 w700 w817 w912 w987 w1044 w1085 w1111] -> w3
    tunnel: w1 -> [w543 w699 w816 w911 w986 w1043 w1084 w1110]
    tunnel: w22 -> [w542 _ _ _ _ _ _ _]
    tunnel: [w542 _ _ _ _ _ _ _] -> w23
    tunnel: [w540 _ _ _ _ _ _ _] -> w20
    tunnel: w8 -> [w538 w696 w814 w908 w984 w1040 w1082 w1109]
    tunnel: [w539 w697 w813 w909 w983 w1041 w1081 w1108] -> w6
    tunnel: [w537 w695 w812 w907 w982 w1039 w1080 w1107] -> w2
    frame 8, Default {
      n263 = for {
        tunnel: w552 -> [w569]
        tunnel: w551 -> [w568]
        tunnel: w550 -> [w567]
        tunnel: w549 -> [w566]
        tunnel: w548 -> [w565]
        tunnel: w547 -> [w564]
        tunnel: w546 -> [w563]
        tunnel: w545 -> [w562] mode=indexing
        shift-right: [w561] -> _
        shift-left: _ -> [_]
        tunnel: [w560] -> w544
        tunnel: w543 -> [w559]
        shift-right: [w557] -> _
        shift-left: 0.0 -> [w558]
        tunnel: [w556] -> w540
        tunnel: [w555] -> w539
        tunnel: w538 -> [w554]
        tunnel: [w553] -> w537 mode=concatenating
        stop <- w556 stop-if-true
        n264 = for {
          tunnel: w569 -> [w586]
          tunnel: w568 -> [w585]
          tunnel: w567 -> [w584]
          tunnel: w566 -> [w583]
          tunnel: w565 -> [w582]
          tunnel: w564 -> [w581]
          tunnel: w563 -> [w580] mode=indexing
          shift-right: [w579] -> w561
          shift-left: _ -> [_]
          tunnel: w562 -> [w578]
          tunnel: [w577] -> w560
          tunnel: w559 -> [w576]
          shift-right: [w574] -> w557
          shift-left: w558 -> [w575]
          tunnel: [w573] -> w556
          tunnel: [w572] -> w555
          tunnel: w554 -> [w571]
          tunnel: [w570] -> w553 mode=concatenating
          stop <- w573 stop-if-true
          n265 = for {
            tunnel: w586 -> [w603]
            tunnel: w585 -> [w602]
            tunnel: w584 -> [w601]
            tunnel: w583 -> [w600]
            tunnel: w582 -> [w599]
            tunnel: w581 -> [w598] mode=indexing
            shift-right: [w597] -> w579
            shift-left: _ -> [_]
            tunnel: w580 -> [w596]
            tunnel: w578 -> [w595]
            tunnel: [w594] -> w577
            tunnel: w576 -> [w593]
            shift-right: [w591] -> w574
            shift-left: w575 -> [w592]
            tunnel: [w590] -> w573
            tunnel: [w589] -> w572
            tunnel: w571 -> [w588]
            tunnel: [w587] -> w570 mode=concatenating
            stop <- w590 stop-if-true
            n266 = for {
              tunnel: w603 -> [w620]
              tunnel: w602 -> [w619]
              tunnel: w601 -> [w618]
              tunnel: w600 -> [w617]
              tunnel: w599 -> [w616] mode=indexing
              shift-right: [w615] -> w597
              shift-left: _ -> [_]
              tunnel: w598 -> [w614]
              tunnel: w596 -> [w613]
              tunnel: w595 -> [w612]
              tunnel: [w611] -> w594
              tunnel: w593 -> [w610]
              shift-right: [w608] -> w591
              shift-left: w592 -> [w609]
              tunnel: [w607] -> w590
              tunnel: [w606] -> w589
              tunnel: w588 -> [w605]
              tunnel: [w604] -> w587 mode=concatenating
              stop <- w607 stop-if-true
              n267 = for {
                tunnel: w620 -> [w637]
                tunnel: w619 -> [w636]
                tunnel: w618 -> [w635]
                tunnel: w617 -> [w634] mode=indexing
                shift-right: [w633] -> w615
                shift-left: _ -> [_]
                tunnel: w616 -> [w632]
                tunnel: w614 -> [w631]
                tunnel: w613 -> [w630]
                tunnel: w612 -> [w629]
                tunnel: [w628] -> w611
                tunnel: w610 -> [w627]
                shift-right: [w625] -> w608
                shift-left: w609 -> [w626]
                tunnel: [w624] -> w607
                tunnel: [w623] -> w606
                tunnel: w605 -> [w622]
                tunnel: [w621] -> w604 mode=concatenating
                stop <- w624 stop-if-true
                n268 = for {
                  tunnel: w637 -> [w654]
                  tunnel: w636 -> [w653]
                  tunnel: w635 -> [w652] mode=indexing
                  shift-right: [w651] -> w633
                  shift-left: _ -> [_]
                  tunnel: w634 -> [w650]
                  tunnel: w632 -> [w649]
                  tunnel: w631 -> [w648]
                  tunnel: w630 -> [w647]
                  tunnel: w629 -> [w646]
                  tunnel: [w645] -> w628
                  tunnel: w627 -> [w644]
                  shift-right: [w642] -> w625
                  shift-left: w626 -> [w643]
                  tunnel: [w641] -> w624
                  tunnel: [w640] -> w623
                  tunnel: w622 -> [w639]
                  tunnel: [w638] -> w621 mode=concatenating
                  stop <- w641 stop-if-true
                  n269 = for {
                    tunnel: w654 -> [w671]
                    shift-right: [w663] -> w651
                    shift-left: _ -> [_]
                    tunnel: w653 -> [w670] mode=indexing
                    tunnel: w652 -> [w669]
                    tunnel: w650 -> [w668]
                    tunnel: w649 -> [w667]
                    tunnel: w648 -> [w666]
                    tunnel: w647 -> [w665]
                    tunnel: w646 -> [w664]
                    tunnel: [w662] -> w645
                    tunnel: w644 -> [w661]
                    shift-right: [w659] -> w642
                    shift-left: w643 -> [w660]
                    tunnel: [w658] -> w641
                    tunnel: [w657] -> w640
                    tunnel: w639 -> [w656]
                    tunnel: [w655] -> w638 mode=concatenating
                    stop <- w658 stop-if-true
                    n270 = for {
                      tunnel: w671 -> [w694] mode=indexing
                      tunnel: w670 -> [w693]
                      tunnel: w669 -> [w692]
                      tunnel: w668 -> [w691]
                      tunnel: w667 -> [w690]
                      tunnel: w666 -> [w689]
                      tunnel: w665 -> [w688]
                      tunnel: w664 -> [w687]
                      tunnel: [w672] -> w663 mode=indexing
                      tunnel: [w673] -> w662
                      tunnel: w661 -> [w673]
                      shift-right: [w677] -> w659
                      shift-left: w660 -> [w684]
                      tunnel: ["STOP TEST"] -> w658
                      tunnel: [w675] -> w657
                      tunnel: w656 -> [w674]
                      tunnel: [w672] -> w655 mode=indexing
                      stop <- "STOP TEST" stop-if-true
                      n271 = Build Array(w694, w693, w692, w691, w690, w689, w688, w687) -> (w686:string[])
                      n272 = Add(x=w684, y=1.0) -> (x+y=w677:dbl)
                      n273 = local write "count"(w677) -> ()
                      n274 = local write "Slide"(w677) -> ()
                      n275 = local read "#of Iterations(str)"() -> (w680:string)
                      n276 = Reverse 1D Array(array=w686) -> (reversed array=w672:string[])
                      n277 = local read "Caption.Text"() -> (w682:string)
                      n278 = Number To Decimal String(number=w677) -> (decimal integer string=w681:string)  [unwired: 1 in]
                      n279 = Concatenate Strings(w682, w681, " of " ("string"), w680, " Iterations" ("string")) -> (w683:string)
                      n280 = property on="Slide" class="Slide (strict)"(error in=w674, "Caption.Text"=w683) -> (error out=w675:errorcluster)  [unwired: 1 in, 1 out]
                    }
                  }
                }
              }
            }
          }
        }
      }
    }
    frame 7 {
      n281 = for {
        tunnel: w707 -> [w722]
        tunnel: w706 -> [w721]
        tunnel: w705 -> [w720]
        tunnel: w704 -> [w719]
        tunnel: w703 -> [w718]
        tunnel: w702 -> [w717]
        shift-right: [w716] -> _
        shift-left: _ -> [_]
        tunnel: w701 -> [w715] mode=indexing
        tunnel: [w714] -> w700
        tunnel: w699 -> [w713]
        shift-right: [w712] -> _
        shift-left: 0.0 -> [w711]
        tunnel: [w710] -> w697
        tunnel: w696 -> [w709]
        tunnel: [w708] -> w695 mode=concatenating
        n282 = for {
          tunnel: w722 -> [w737]
          tunnel: w721 -> [w736]
          tunnel: w720 -> [w735]
          tunnel: w719 -> [w734]
          tunnel: w718 -> [w733]
          shift-right: [w732] -> w716
          shift-left: _ -> [_]
          tunnel: w717 -> [w731] mode=indexing
          tunnel: w715 -> [w730]
          tunnel: [w729] -> w714
          tunnel: w713 -> [w728]
          shift-right: [w726] -> w712
          shift-left: w711 -> [w727]
          tunnel: [w725] -> w710
          tunnel: w709 -> [w724]
          tunnel: [w723] -> w708 mode=concatenating
          n283 = for {
            tunnel: w737 -> [w752]
            tunnel: w736 -> [w751]
            tunnel: w735 -> [w750]
            tunnel: w734 -> [w749]
            shift-right: [w748] -> w732
            shift-left: _ -> [_]
            tunnel: w733 -> [w747] mode=indexing
            tunnel: w731 -> [w746]
            tunnel: w730 -> [w745]
            tunnel: [w744] -> w729
            tunnel: w728 -> [w743]
            shift-right: [w741] -> w726
            shift-left: w727 -> [w742]
            tunnel: [w740] -> w725
            tunnel: w724 -> [w739]
            tunnel: [w738] -> w723 mode=concatenating
            n284 = for {
              tunnel: w752 -> [w767]
              tunnel: w751 -> [w766]
              tunnel: w750 -> [w765]
              shift-right: [w764] -> w748
              shift-left: _ -> [_]
              tunnel: w749 -> [w763] mode=indexing
              tunnel: w747 -> [w762]
              tunnel: w746 -> [w761]
              tunnel: w745 -> [w760]
              tunnel: [w759] -> w744
              tunnel: w743 -> [w758]
              shift-right: [w756] -> w741
              shift-left: w742 -> [w757]
              tunnel: [w755] -> w740
              tunnel: w739 -> [w754]
              tunnel: [w753] -> w738 mode=concatenating
              n285 = for {
                tunnel: w767 -> [w782]
                tunnel: w766 -> [w781]
                shift-right: [w780] -> w764
                shift-left: _ -> [_]
                tunnel: w765 -> [w779] mode=indexing
                tunnel: w763 -> [w778]
                tunnel: w762 -> [w777]
                tunnel: w761 -> [w776]
                tunnel: w760 -> [w775]
                tunnel: [w774] -> w759
                tunnel: w758 -> [w773]
                shift-right: [w771] -> w756
                shift-left: w757 -> [w772]
                tunnel: [w770] -> w755
                tunnel: w754 -> [w769]
                tunnel: [w768] -> w753 mode=concatenating
                n286 = for {
                  shift-right: [w790] -> w780
                  shift-left: _ -> [_]
                  tunnel: w782 -> [w797]
                  tunnel: w781 -> [w796] mode=indexing
                  tunnel: w779 -> [w795]
                  tunnel: w778 -> [w794]
                  tunnel: w777 -> [w793]
                  tunnel: w776 -> [w792]
                  tunnel: w775 -> [w791]
                  tunnel: [w789] -> w774
                  tunnel: w773 -> [w788]
                  shift-right: [w786] -> w771
                  shift-left: w772 -> [w787]
                  tunnel: [w785] -> w770
                  tunnel: w769 -> [w784]
                  tunnel: [w783] -> w768 mode=concatenating
                  n287 = for {
                    tunnel: w797 -> [w811] mode=indexing
                    tunnel: w796 -> [w810]
                    tunnel: w795 -> [w809]
                    tunnel: w794 -> [w808]
                    tunnel: w793 -> [w807]
                    tunnel: w792 -> [w806]
                    tunnel: w791 -> [w805]
                    tunnel: [w798] -> w790 mode=indexing
                    tunnel: [w799] -> w789
                    tunnel: w788 -> [w799]
                    shift-right: [w801] -> w786
                    shift-left: w787 -> [w802]
                    tunnel: [w800] -> w785
                    tunnel: w784 -> [w800]
                    tunnel: [w798] -> w783 mode=indexing
                    n288 = Build Array(w811, w810, w809, w808, w807, w806, w805) -> (w804:string[])
                    n289 = Add(x=w802, y=1.0) -> (x+y=w801:dbl)
                    n290 = local write "count"(w801) -> ()
                    n291 = Reverse 1D Array(array=w804) -> (reversed array=w798:string[])
                  }
                }
              }
            }
          }
        }
      }
    }
    frame 6 {
      n292 = for {
        tunnel: w823 -> [w837]
        tunnel: w822 -> [w836]
        tunnel: w821 -> [w835]
        tunnel: w820 -> [w834]
        shift-right: [w833] -> _
        shift-left: _ -> [_]
        tunnel: w819 -> [w832]
        tunnel: w818 -> [w831] mode=indexing
        tunnel: [w830] -> w817
        tunnel: w816 -> [w829]
        shift-right: [w827] -> _
        shift-left: 0.0 -> [w828]
        tunnel: w814 -> [w826]
        tunnel: [w825] -> w813
        tunnel: [w824] -> w812 mode=concatenating
        n293 = for {
          tunnel: w837 -> [w851]
          tunnel: w836 -> [w850]
          tunnel: w835 -> [w849]
          shift-right: [w848] -> w833
          shift-left: _ -> [_]
          tunnel: w834 -> [w847]
          tunnel: w832 -> [w846] mode=indexing
          tunnel: w831 -> [w845]
          tunnel: [w844] -> w830
          tunnel: w829 -> [w843]
          shift-right: [w841] -> w827
          shift-left: w828 -> [w842]
          tunnel: w826 -> [w840]
          tunnel: [w839] -> w825
          tunnel: [w838] -> w824 mode=concatenating
          n294 = for {
            tunnel: w851 -> [w865]
            tunnel: w850 -> [w864]
            shift-right: [w863] -> w848
            shift-left: _ -> [_]
            tunnel: w849 -> [w862]
            tunnel: w847 -> [w861] mode=indexing
            tunnel: w846 -> [w860]
            tunnel: w845 -> [w859]
            tunnel: [w858] -> w844
            tunnel: w843 -> [w857]
            shift-right: [w855] -> w841
            shift-left: w842 -> [w856]
            tunnel: w840 -> [w854]
            tunnel: [w853] -> w839
            tunnel: [w852] -> w838 mode=concatenating
            n295 = for {
              tunnel: w865 -> [w879]
              shift-right: [w878] -> w863
              shift-left: _ -> [_]
              tunnel: w864 -> [w877]
              tunnel: w862 -> [w876] mode=indexing
              tunnel: w861 -> [w875]
              tunnel: w860 -> [w874]
              tunnel: w859 -> [w873]
              tunnel: [w872] -> w858
              tunnel: w857 -> [w871]
              shift-right: [w869] -> w855
              shift-left: w856 -> [w870]
              tunnel: w854 -> [w868]
              tunnel: [w867] -> w853
              tunnel: [w866] -> w852 mode=concatenating
              n296 = for {
                shift-right: [w887] -> w878
                shift-left: _ -> [_]
                tunnel: w879 -> [w893]
                tunnel: w877 -> [w892] mode=indexing
                tunnel: w876 -> [w891]
                tunnel: w875 -> [w890]
                tunnel: w874 -> [w889]
                tunnel: w873 -> [w888]
                tunnel: [w886] -> w872
                tunnel: w871 -> [w885]
                shift-right: [w883] -> w869
                shift-left: w870 -> [w884]
                tunnel: w868 -> [w882]
                tunnel: [w881] -> w867
                tunnel: [w880] -> w866 mode=concatenating
                n297 = for {
                  tunnel: w893 -> [w906] mode=indexing
                  tunnel: w892 -> [w905]
                  tunnel: w891 -> [w904]
                  tunnel: w890 -> [w903]
                  tunnel: w889 -> [w902]
                  tunnel: w888 -> [w901]
                  tunnel: [w894] -> w887 mode=indexing
                  tunnel: [w895] -> w886
                  tunnel: w885 -> [w895]
                  shift-right: [w897] -> w883
                  shift-left: w884 -> [w898]
                  tunnel: w882 -> [w896]
                  tunnel: [w896] -> w881
                  tunnel: [w894] -> w880 mode=indexing
                  n298 = Build Array(w906, w905, w904, w903, w902, w901) -> (w900:string[])
                  n299 = Add(x=w898, y=1.0) -> (x+y=w897:dbl)
                  n300 = local write "count"(w897) -> ()
                  n301 = Reverse 1D Array(array=w900) -> (reversed array=w894:string[])
                }
              }
            }
          }
        }
      }
    }
    frame 5 {
      n302 = for {
        tunnel: w917 -> [w930]
        tunnel: w916 -> [w929]
        shift-right: [w928] -> _
        shift-left: _ -> [_]
        tunnel: w915 -> [w927]
        tunnel: w914 -> [w926]
        tunnel: w913 -> [w925] mode=indexing
        tunnel: [w924] -> w912
        tunnel: w911 -> [w923]
        shift-right: [w921] -> _
        shift-left: 0.0 -> [w922]
        tunnel: [w920] -> w909
        tunnel: w908 -> [w919]
        tunnel: [w918] -> w907 mode=concatenating
        n303 = for {
          tunnel: w930 -> [w943]
          shift-right: [w942] -> w928
          shift-left: _ -> [_]
          tunnel: w929 -> [w941]
          tunnel: w927 -> [w940]
          tunnel: w926 -> [w939] mode=indexing
          tunnel: w925 -> [w938]
          tunnel: [w937] -> w924
          tunnel: w923 -> [w936]
          shift-right: [w934] -> w921
          shift-left: w922 -> [w935]
          tunnel: [w933] -> w920
          tunnel: w919 -> [w932]
          tunnel: [w931] -> w918 mode=concatenating
          n304 = for {
            shift-right: [w956] -> w942
            shift-left: _ -> [_]
            tunnel: w943 -> [w955]
            tunnel: w941 -> [w954]
            tunnel: w940 -> [w953] mode=indexing
            tunnel: w939 -> [w952]
            tunnel: w938 -> [w951]
            tunnel: [w950] -> w937
            tunnel: w936 -> [w949]
            shift-right: [w948] -> w934
            shift-left: w935 -> [w947]
            tunnel: [w946] -> w933
            tunnel: w932 -> [w945]
            tunnel: [w944] -> w931 mode=concatenating
            n305 = for {
              shift-right: [w964] -> w956
              shift-left: _ -> [_]
              tunnel: w955 -> [w969]
              tunnel: w954 -> [w968] mode=indexing
              tunnel: w953 -> [w967]
              tunnel: w952 -> [w966]
              tunnel: w951 -> [w965]
              tunnel: [w963] -> w950
              tunnel: w949 -> [w962]
              shift-right: [w961] -> w948
              shift-left: w947 -> [w960]
              tunnel: [w959] -> w946
              tunnel: w945 -> [w958]
              tunnel: [w957] -> w944 mode=concatenating
              n306 = for {
                tunnel: w969 -> [w981] mode=indexing
                tunnel: w968 -> [w980]
                tunnel: w967 -> [w979]
                tunnel: w966 -> [w978]
                tunnel: w965 -> [w977]
                tunnel: [w970] -> w964 mode=indexing
                tunnel: [w972] -> w963
                tunnel: w962 -> [w972]
                shift-right: [w973] -> w961
                shift-left: w960 -> [w974]
                tunnel: [w971] -> w959
                tunnel: w958 -> [w971]
                tunnel: [w970] -> w957 mode=indexing
                n307 = Build Array(w981, w980, w979, w978, w977) -> (w976:string[])
                n308 = Add(x=w974, y=1.0) -> (x+y=w973:dbl)
                n309 = local write "count"(w973) -> ()
                n310 = Reverse 1D Array(array=w976) -> (reversed array=w970:string[])
              }
            }
          }
        }
      }
    }
    frame 4 {
      n311 = for {
        shift-right: [w1003] -> _
        shift-left: _ -> [_]
        tunnel: w991 -> [w1002]
        tunnel: w990 -> [w1001]
        tunnel: w989 -> [w1000]
        tunnel: w988 -> [w999] mode=indexing
        tunnel: [w998] -> w987
        tunnel: w986 -> [w997]
        shift-right: [w995] -> _
        shift-left: 0.0 -> [w996]
        tunnel: w984 -> [w994]
        tunnel: [w993] -> w983
        tunnel: [w992] -> w982 mode=concatenating
        n312 = for {
          shift-right: [w1015] -> w1003
          shift-left: _ -> [_]
          tunnel: w1002 -> [w1014]
          tunnel: w1001 -> [w1013]
          tunnel: w1000 -> [w1012] mode=indexing
          tunnel: w999 -> [w1011]
          tunnel: [w1010] -> w998
          tunnel: w997 -> [w1009]
          shift-right: [w1007] -> w995
          shift-left: w996 -> [w1008]
          tunnel: w994 -> [w1006]
          tunnel: [w1005] -> w993
          tunnel: [w1004] -> w992 mode=concatenating
          n313 = for {
            shift-right: [w1023] -> w1015
            shift-left: _ -> [_]
            tunnel: w1014 -> [w1027]
            tunnel: w1013 -> [w1026] mode=indexing
            tunnel: w1012 -> [w1025]
            tunnel: w1011 -> [w1024]
            tunnel: [w1022] -> w1010
            tunnel: w1009 -> [w1021]
            shift-right: [w1019] -> w1007
            shift-left: w1008 -> [w1020]
            tunnel: w1006 -> [w1018]
            tunnel: [w1017] -> w1005
            tunnel: [w1016] -> w1004 mode=concatenating
            n314 = for {
              tunnel: w1027 -> [w1038] mode=indexing
              tunnel: w1026 -> [w1037]
              tunnel: w1025 -> [w1036]
              tunnel: w1024 -> [w1035]
              tunnel: [w1028] -> w1023 mode=indexing
              tunnel: [w1029] -> w1022
              tunnel: w1021 -> [w1029]
              shift-right: [w1033] -> w1019
              shift-left: w1020 -> [w1032]
              tunnel: w1018 -> [w1030]
              tunnel: [w1030] -> w1017
              tunnel: [w1028] -> w1016 mode=indexing
              n315 = Build Array(w1038, w1037, w1036, w1035) -> (w1034:string[])
              n316 = Add(x=w1032, y=1.0) -> (x+y=w1033:dbl)
              n317 = local write "count"(w1033) -> ()
              n318 = Reverse 1D Array(array=w1034) -> (reversed array=w1028:string[])
            }
          }
        }
      }
    }
    frame 3 {
      n319 = for {
        shift-right: [w1058] -> _
        shift-left: _ -> [_]
        tunnel: w1047 -> [w1057]
        tunnel: w1046 -> [w1056]
        tunnel: w1045 -> [w1055] mode=indexing
        tunnel: [w1054] -> w1044
        tunnel: w1043 -> [w1053]
        shift-right: [w1051] -> _
        shift-left: 0.0 -> [w1052]
        tunnel: [w1050] -> w1041
        tunnel: w1040 -> [w1049]
        tunnel: [w1048] -> w1039 mode=concatenating
        n320 = for {
          shift-right: [w1066] -> w1058
          shift-left: _ -> [_]
          tunnel: w1057 -> [w1069]
          tunnel: w1056 -> [w1068] mode=indexing
          tunnel: w1055 -> [w1067]
          tunnel: [w1065] -> w1054
          tunnel: w1053 -> [w1064]
          shift-right: [w1062] -> w1051
          shift-left: w1052 -> [w1063]
          tunnel: [w1061] -> w1050
          tunnel: w1049 -> [w1060]
          tunnel: [w1059] -> w1048 mode=concatenating
          n321 = for {
            tunnel: w1069 -> [w1079] mode=indexing
            tunnel: w1068 -> [w1078]
            tunnel: w1067 -> [w1077]
            tunnel: [w1070] -> w1066 mode=indexing
            tunnel: [w1072] -> w1065
            tunnel: w1064 -> [w1072]
            shift-right: [w1073] -> w1062
            shift-left: w1063 -> [w1074]
            tunnel: [w1071] -> w1061
            tunnel: w1060 -> [w1071]
            tunnel: [w1070] -> w1059 mode=indexing
            n322 = Build Array(w1079, w1078, w1077) -> (w1076:string[])
            n323 = Add(x=w1074, y=1.0) -> (x+y=w1073:dbl)
            n324 = local write "count"(w1073) -> ()
            n325 = Reverse 1D Array(array=w1076) -> (reversed array=w1070:string[])
          }
        }
      }
    }
    frame 2 {
      n326 = for {
        shift-right: [w1095] -> _
        shift-left: _ -> [_]
        tunnel: w1087 -> [w1097]
        tunnel: w1086 -> [w1096] mode=indexing
        tunnel: [w1094] -> w1085
        tunnel: w1084 -> [w1093]
        shift-right: [w1091] -> _
        shift-left: 0.0 -> [w1092]
        tunnel: w1082 -> [w1090]
        tunnel: [w1089] -> w1081
        tunnel: [w1088] -> w1080 mode=concatenating
        n327 = for {
          tunnel: w1097 -> [w1106] mode=indexing
          tunnel: w1096 -> [w1105]
          tunnel: [w1098] -> w1095 mode=indexing
          tunnel: [w1099] -> w1094
          tunnel: w1093 -> [w1099]
          shift-right: [w1101] -> w1091
          shift-left: w1092 -> [w1103]
          tunnel: w1090 -> [w1100]
          tunnel: [w1100] -> w1089
          tunnel: [w1098] -> w1088 mode=indexing
          n328 = Build Array(w1106, w1105) -> (w1104:string[])
          n329 = Add(x=w1103, y=1.0) -> (x+y=w1101:dbl)
          n330 = local write "count"(w1101) -> ()
          n331 = Reverse 1D Array(array=w1104) -> (reversed array=w1098:string[])
        }
      }
    }
    frame 1 {
      n332 = for {
        tunnel: w1112 -> [w1118] mode=indexing
        tunnel: [w1117] -> w1107 mode=indexing
        tunnel: [w1113] -> w1111
        tunnel: w1110 -> [w1113]
        tunnel: w1109 -> [w1114]
        tunnel: [w1114] -> w1108
        i -> [w1116]
        n333 = Build Array(w1118) -> (w1117:string[])
        n334 = Increment(x=w1116) -> (x+1=→"count":i32)
      }
    }
  }
  n335 = Concatenate Strings(w39, "Iterations" ("string")) -> (w37:string)
  n336 = Insert Into Array(array=w65, index=w64, new element=w37) -> (w40:string[])
  "Loop Info" <- w40
  n337 = global write "Test Parameter Globals_1.0.0.vi" "Loop Info"(w40) -> ()
  n338 = call <vilib>:"High Resolution Relative Seconds.vi"() -> ("relative seconds"=w24:dbl)
  n339 = case shown="True" w20 {
    selector: w20 -> [_ w1120]
    tunnel: w20 -> [_ w1123]
    tunnel: w6 -> [w1119 w1122]
    tunnel: [w1119 w1121] -> w7
    frame False {
    }
    frame True {
      n340 = global write "Sequence Globals.vi" "Stop Testing"(w1120) -> ()
      n341 = flat-sequence {
        tunnel: w1123 -> [w1127]
        tunnel: [w1127] -> w1124
        tunnel: w1122 -> [w1126]
        tunnel: [w1125] -> w1121
        tunnel: w1124 -> [w1129]
        frame #0 {
          n342 = control-ref of="This VI"() -> (w1128:refnum<vi>)
          n343 = invoke class="VI" method="FP.Close"(reference=w1128, error in=w1126) -> (error out=w1125:errorcluster)  [unwired: 1 in, 2 out]
        }
        frame #1 {
          n344 = Stop(stop? (T)=w1129) -> ()
        }
      }
    }
  }
  "error out" <- w7
  n345 = call-poly <vilib>:"Write Delimited Spreadsheet.vi"("file path (dialog if empty)"=w3, "2D data"=w2, "append to file? (new file:F)"=TRUE, "delimiter (\\t)"="," ("delimiter (\\t)")) -> ()  [unwired: 10 in, 2 out]
  n346 = Subtract(x=w24, y=w23) -> (x-y=→"x-y 13":dbl)
